vi "Graphing Data (global).vi"(0 "Title IN":string, 1 "Main Side IN":bool, 2 "Wet Test IN":bool, 3 "Y-Axis Max IN":i32, 4 "Data End Index IN":i32, 5 "MLS Test IN":bool, 6 "Data Base Path IN":path, 7 "Tolerances Path IN":path, 8 "File Name IN":string, 9 "Python Script Directory IN":path=path "C:/Users/gtetil/Documents/Projects/ls-tester-graph-script", 10 "Graph Settings IN":T1, 11 "Data Start Index IN":u32, 12 "Mode":enum16{"Read", "Write", "Init", "Stop"}(ring)) -> (14 "Graph Settings OUT":T1, 15 "STOP":bool, 16 "Data Ready?":bool, 17 "Data Start Index":u32, 18 "File Name":string, 19 "Python Script Directory":path, 20 "Title":string, 21 "Main Side":bool, 22 "Wet Test":bool, 23 "Y-Axis Max":i32, 24 "Data End Index":i32, 25 "MLS Test":bool, 26 "Data Base Path":path, 27 "Tolerances Path":path)   [LabVIEW 2013]
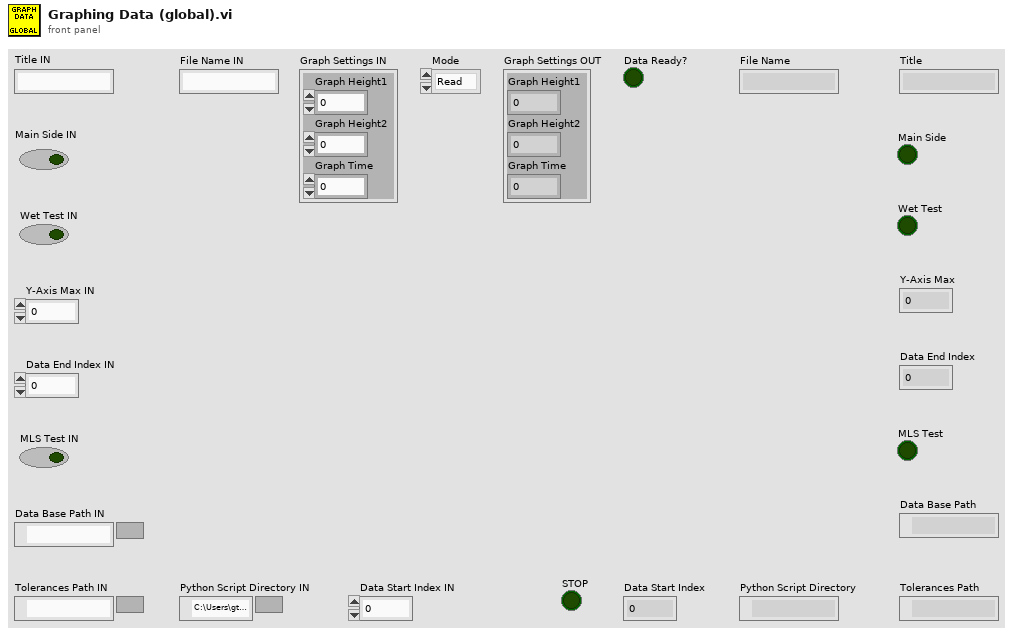
[diagram p1: front panel]
types:
  T1 = cluster{"Graph Height1":dbl, "Graph Height2":dbl, "Graph Time":dbl}
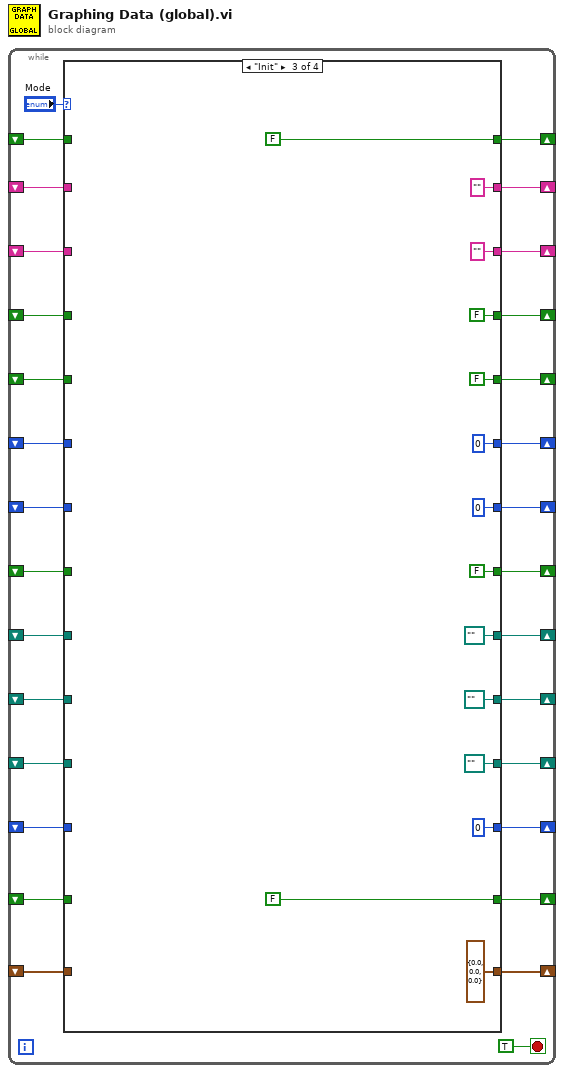
[diagram p0: block diagram]
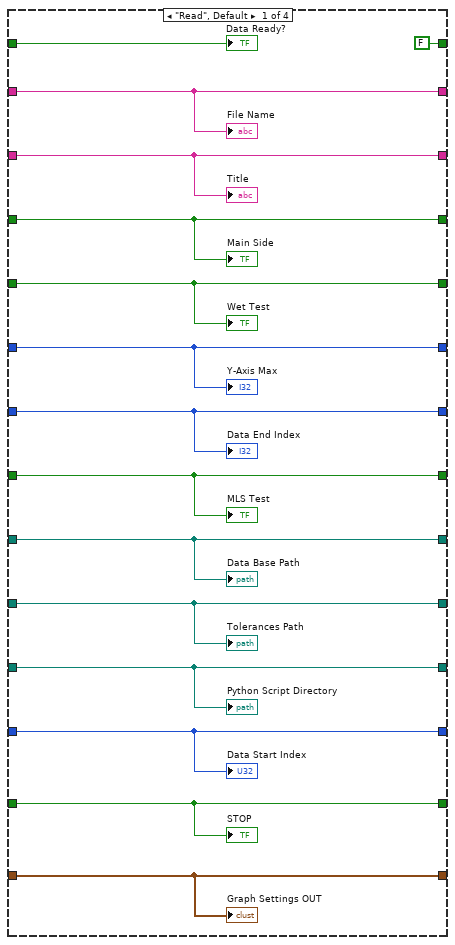
[diagram p2: hidden frame]
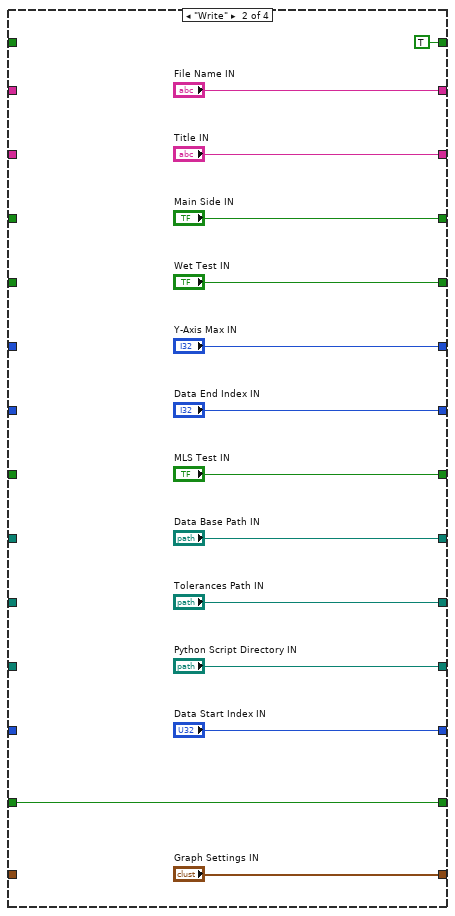
[diagram p3: hidden frame]
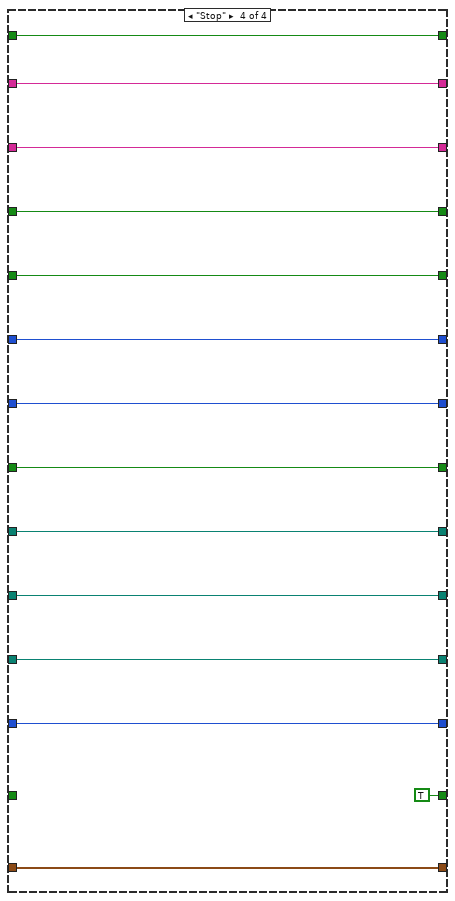
[diagram p4: hidden frame]
diagram:
  n1 = while {
    shift-right: [w18] -> _
    shift-left: _ -> [w5]
    shift-right: [w19] -> _
    shift-left: _ -> [w6]
    shift-right: [w20] -> _
    shift-left: _ -> [w7]
    shift-right: [w21] -> _
    shift-left: _ -> [w8]
    shift-right: [w22] -> _
    shift-left: _ -> [w9]
    shift-right: [w23] -> _
    shift-left: _ -> [w10]
    shift-right: [w24] -> _
    shift-left: _ -> [w11]
    shift-right: [w25] -> _
    shift-left: _ -> [w12]
    shift-right: [w26] -> _
    shift-left: _ -> [w13]
    shift-right: [w27] -> _
    shift-left: _ -> [w14]
    shift-right: [w28] -> _
    shift-left: _ -> [w15]
    shift-right: [w17] -> _
    shift-left: _ -> [w16]
    shift-right: [w4] -> _
    shift-left: _ -> [w3]
    shift-right: [w2] -> _
    shift-left: _ -> [w1]
    stop <- TRUE stop-if-true
    n2 = case shown="\"Init\"" "Mode" {
      tunnel: [w35 "File Name IN" "" ("File Name") w86] -> w28
      tunnel: [w36 "Title IN" "" ("Title") w85] -> w27
      tunnel: [w37 "Main Side IN" FALSE ("Main Side") w84] -> w26
      tunnel: [w38 "Wet Test IN" FALSE ("Wet Test") w83] -> w25
      tunnel: [w39 "Y-Axis Max IN" 0 ("Y-Axis Max") w82] -> w24
      tunnel: [w40 "Data End Index IN" 0 ("Data End Index") w81] -> w23
      tunnel: [w41 "MLS Test IN" FALSE ("MLS Test") w80] -> w22
      tunnel: [w42 "Data Base Path IN" path "" ("Data Base Path") w79] -> w21
      tunnel: [w43 "Tolerances Path IN" path "" ("Tolerances Path") w78] -> w20
      tunnel: [w44 "Python Script Directory IN" path "" ("Python Script Directory") w77] -> w19
      tunnel: [w45 "Data Start Index IN" u32 0 ("Data Start Index") w76] -> w18
      tunnel: [FALSE TRUE FALSE w87] -> w17
      tunnel: w16 -> [w33 _ _ w87]
      tunnel: w15 -> [w35 _ _ w86]
      tunnel: w14 -> [w36 _ _ w85]
      tunnel: w13 -> [w37 _ _ w84]
      tunnel: w12 -> [w38 _ _ w83]
      tunnel: w11 -> [w39 _ _ w82]
      tunnel: w10 -> [w40 _ _ w81]
      tunnel: w9 -> [w41 _ _ w80]
      tunnel: w8 -> [w42 _ _ w79]
      tunnel: w7 -> [w43 _ _ w78]
      tunnel: w6 -> [w44 _ _ w77]
      tunnel: w5 -> [w45 _ _ w76]
      tunnel: [w32 w47 FALSE TRUE] -> w4
      tunnel: w3 -> [w32 w47 _ _]
      tunnel: [w31 "Graph Settings IN" T1 {"Graph Height1"=0.0, "Graph Height2"=0.0, "Graph Time"=0.0} ("Graph Settings IN") w74] -> w2
      tunnel: w1 -> [w31 _ _ w74]
      frame "Read", Default {
        "File Name" <- w35
        "Data Ready?" <- w33
        "Title" <- w36
        "Main Side" <- w37
        "Wet Test" <- w38
        "Y-Axis Max" <- w39
        "Data End Index" <- w40
        "MLS Test" <- w41
        "Data Base Path" <- w42
        "Tolerances Path" <- w43
        "Python Script Directory" <- w44
        "Data Start Index" <- w45
        "STOP" <- w32
        "Graph Settings OUT" <- w31
      }
      frame "Write" {
      }
      frame "Init" {
      }
      frame "Stop" {
      }
    }
  }
